vi "Camera_Grab.vi"(8 "error in":errorcluster, 11 "Session In":T3="cam1") -> (0 "error out":errorcluster, 3 "Image":T2(plugin-control))   [LabVIEW 2023]
doc: "Vi qui permet d'afficher en live les images d'une caméra (webcam) et qui permet de sauver une image à un moment donné dans un fichier png"
uses:
  <vilib>/vision/driver/NI_Vision_Acquisition_Software.lvlib
  <vilib>/userDefined/High Color/IMAQdx.ctl
panel:
  in  "Saving parameters":T1={"Path on the output file"=path "D:/Programmation/Labview_ILM_LIDT/DATA", "Filename without extension"="Measurement_1"}
  in  "Menu":string(combo)="---"
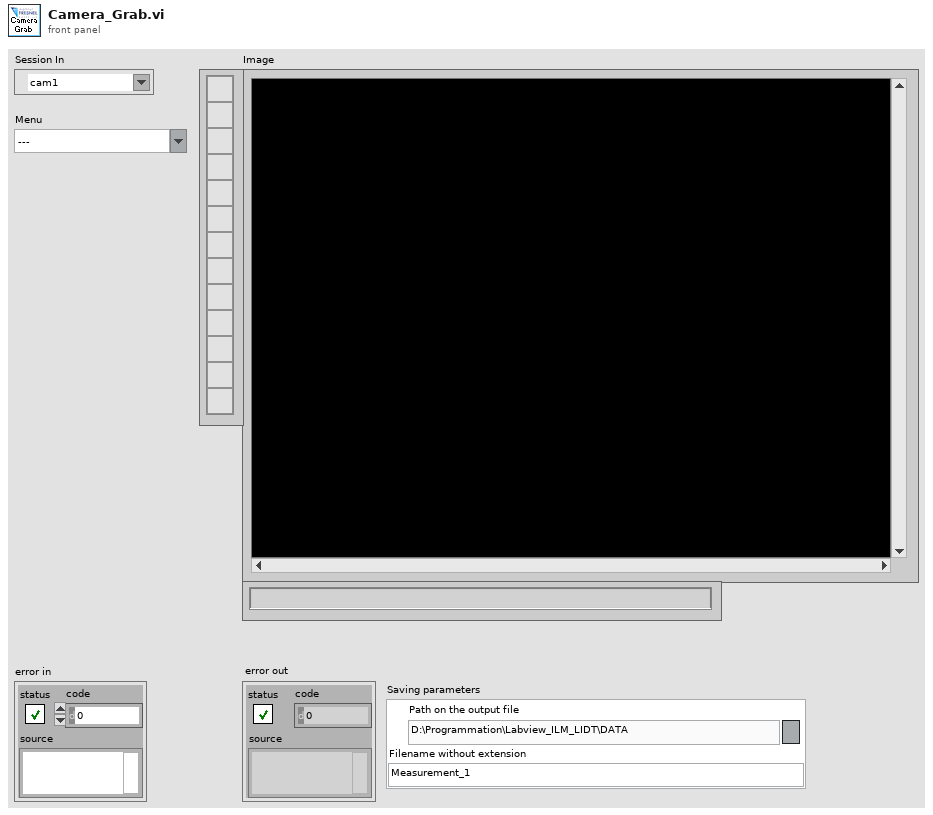
[diagram p1: front panel]
types:
  T1 = cluster{"Path on the output file":path, "Filename without extension":string}
  T2 = typedef "IMAQ Image.ctl" = refnum<image>
  T3 = typedef "IMAQdx.ctl" = refnum<k21>
  T4 = typedef "Image Type" = u32
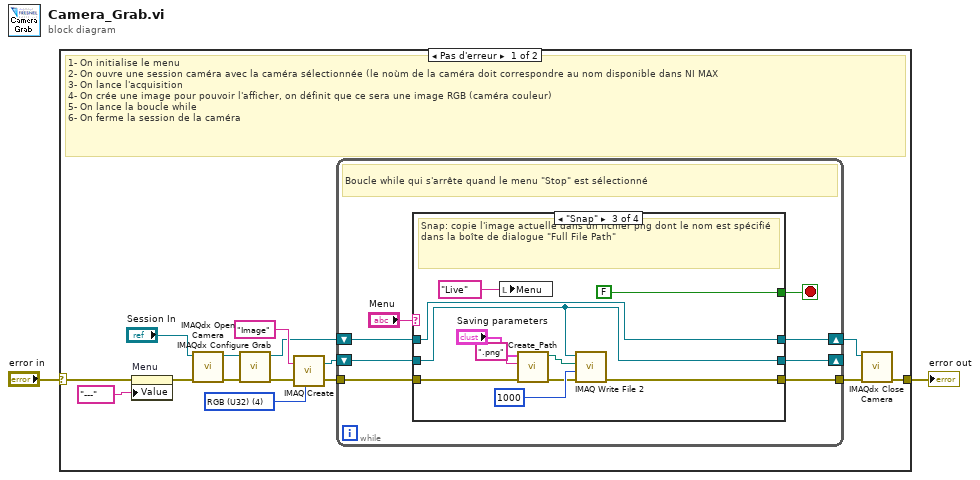
[diagram p0: block diagram]
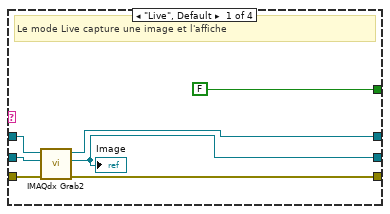
[diagram p2: hidden frame]
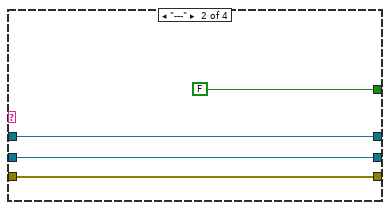
[diagram p3: hidden frame]
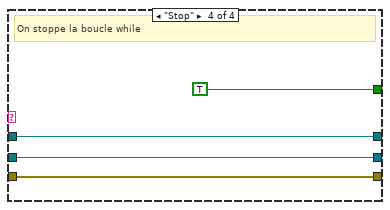
[diagram p4: hidden frame]
diagram:
  n1 = case shown="Pas d'erreur" "error in" {
    selector: "error in" -> [w5 w52]
    tunnel: [w11 w52] -> w2
    frame No Error {
      w12 = T4 4 items=["Grayscale (U8)", "Grayscale (I16)", "Grayscale (SGL)", "Complex (CSG)", "RGB (U32)", "HSL (U32)", "RGB (U64)", "Grayscale (U16)"] ("Image Type")
      # "1- On initialise le menu\n2- On ouvre une session caméra avec la caméra sélectionnée (le noùm de la caméra doit correspondre au nom disponible dans NI MAX\n3- On lance l'acquisition\n4- On crée une image pour pouvoir l'afficher, on définit que ce sera une image RGB (caméra couleur)\n5- On lance la boucle while\n6- On ferme la session de la caméra"
      n2 = property on="Menu" class="ChneDér"(error in=w5, "Value"="---" ("Menu")) -> (error out=w4:errorcluster)  [unwired: 1 in, 1 out]
      n3 = call <vilib>:"IMAQdx Open Camera.vi"("error in"=w4, "Session In"="Session In") -> ("error out"=w15:errorcluster, "Session Out"=w16:T3)  [unwired: 8 in]
      n4 = call <vilib>:"IMAQdx Configure Grab.vi"("error in"=w15, "Session In"=w16) -> ("error out"=w17:errorcluster, "Session Out"=w8:T3)  [unwired: 8 in]
      n5 = call "IMAQ Create"("Image Name"="Image", "Image Type"=w12, "error in (no error)"=w17) -> ("New Image"=w9:T2, "error out"=w10:errorcluster)  [unwired: 2 in]
      n6 = while {
        tunnel: w10 -> [w24]
        tunnel: [w23] -> w7
        shift-right: [w19] -> _
        shift-left: w9 -> [w20]
        shift-right: [w21] -> w6
        shift-left: w8 -> [w22]
        stop <- w25 stop-if-true
        # "Boucle while qui s'arrête quand le menu \"Stop\" est sélectionné"
        n7 = case shown="\"Snap\"" "Menu" {
          tunnel: [FALSE ("stop") FALSE ("stop") FALSE ("stop") TRUE ("stop")] -> w25
          tunnel: w24 -> [w31 w35 w39 w51]
          tunnel: [w30 w35 w44 w51] -> w23
          tunnel: w22 -> [w29 w33 w46 w49]
          tunnel: w20 -> [w28 w34 w45 w50]
          tunnel: [w27 w33 w46 w49] -> w21
          tunnel: [w26 w34 w45 w50] -> w19
          frame "Live", Default {
            # "Le mode Live capture une image et l'affiche"
            n8 = call <vilib>:"IMAQdx Grab2.vi"("error in"=w31, "Image In"=w28, "Session In"=w29) -> ("error out"=w30:errorcluster, "Image Out"=w26:T2, "Session Out"=w27:T3)  [unwired: 5 in, 1 out]
            "Image" <- w26
          }
          frame "---" {
          }
          frame "Snap" {
            # "Snap: copie l'image actuelle dans un fichier png dont le nom est spécifié dans la boîte de dialogue \"Full File Path\""
            n9 = local write "Menu"("Live" ("Menu")) -> ()
            n10 = call "Create_Path.vi"("error in"=w39, "Extension"=".png", "Saving parameters"="Saving parameters") -> ("error out"=w38:errorcluster, "File path"=w37:path)  [unwired: 7 in]
            n11 = call-poly "IMAQ Write File 2"("error in (no error)"=w38, "Image Quality"=u32 1000, "File Path"=w37, "Image"=w45) -> ("error out"=w44:errorcluster)  [unwired: 6 in, 1 out]
          }
          frame "Stop" {
            # "On stoppe la boucle while"
          }
        }
      }
      n12 = call <vilib>:"IMAQdx Close Camera.vi"("error in"=w7, "Session In"=w6) -> ("error out"=w11:errorcluster)  [unwired: 9 in]
    }
    frame Error {
    }
  }
  "error out" <- w2
